vi "Read Type-Specific Macro Parameters.vi"(7 "Section":string, 8 "error in (no error)":errorcluster, 10 "Macro Step":T1, 11 "refnum":T5) -> (0 "error out":errorcluster, 2 "Macro Step out":T1={"Type"=enum."Mouse Move", "X"=0, "Y"=0, "Delay"=0, "Key"=65, "Repeat"=0, "RClick?"=FALSE, "App/Window Name"="", "Notes"="", "Assertion Type"=enum."Control Position", "Control Name"="", "Disabled"=enum."Enabled", "Visible"=enum."Visible", "Left"=0, "Top"=0, "Width"=0, "Height"=0, "Expected Image"={"image type"=0, "image depth"=0, "image"=[], "mask"=[], "colors"=[], "Rectangle"={"left"=0, "top"=0, "right"=0, "bottom"=0}}}, 3 "refnum out":T5)   [LabVIEW 2020, in "MacroAssert.lvlib"]
doc: "Reads the list of steps from macro config file defined by <B>refnum</B>."
uses:
  MacroAssert.lvlib
  <vilib>/ErrorRing/Error Ring.xnode
  <vilib>/Utility/config.llb/NI_LVConfig.lvlib
  <vilib>/Utility/config.llb/Read Key (String).vi
  <vilib>/Utility/config.llb/Read Key (I32).vi
  CTLs/Assertion Type.ctl
  <vilib>/Utility/error.llb/Error Cluster From Error Code.vi
  <vilib>/Utility/config.llb/Read Key (Boolean).vi
  <vilib>/Utility/config.llb/Read Key (U32).vi
  <vilib>/Utility/config.llb/Config Data RefNum.ctl
  CTLs/Step Type V3.ctl
  CTLs/Step V3.ctl
  <vilib>/picture/picture.llb/imagedata.ctl
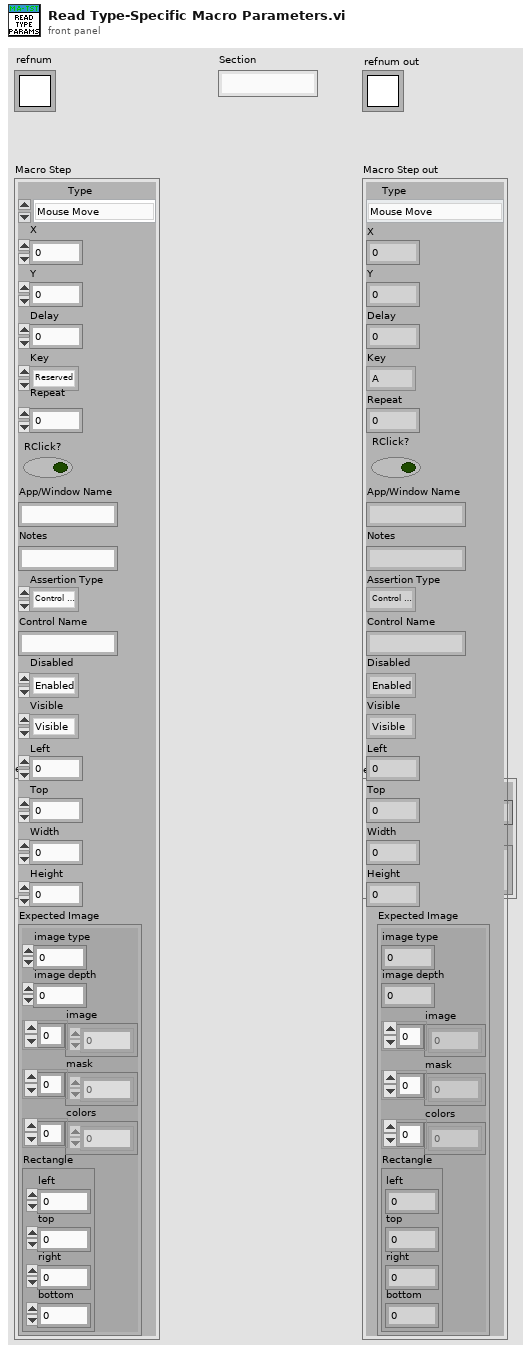
[diagram p1: front panel]
types:
  T1 = typedef "MacroAssert.lvlib/Step V3.ctl" = cluster{"Type":T2, "X":i32, "Y":i32, "Delay":i32, "Key":u8, "Repeat":i32, "RClick?":bool, "App/Window Name":string, "Notes":string, "Assertion Type":T3, "Control Name":string, "Disabled":enum8{"Enabled", "Disabled", "Disabled and Grayed Out"}, "Visible":enum16{"Visible", "Not Visible"}, "Left":i16, "Top":i16, "Width":i16, "Height":i16, "Expected Image":T4}
  T2 = typedef "MacroAssert.lvlib/Step Type V3.ctl" = enum16{"Mouse Move", "Mouse Click", "Key Press", "Wait", "Mouse Down", "Mouse Up", "Key Down", "Key Up", "Test Assertion", "Run Application", "Maximize Window", "Restore Window", "Minimize Window", "Close Window", "Bring Window to Front", "Send Window to Back"}
  T3 = typedef "MacroAssert.lvlib/Assertion Type.ctl" = enum16{"Control Position", "Control Visible", "Control Disabled", "Control Image"}
  T4 = typedef "imagedata.ctl" = cluster{"image type":i32, "image depth":i32, "image":u8[], "mask":u8[], "colors":u32[], "Rectangle":cluster{"left":i16, "top":i16, "right":i16, "bottom":i16}}
  T5 = typedef "NI_LVConfig.lvlib/Config Data RefNum.ctl" = refnum<k1>
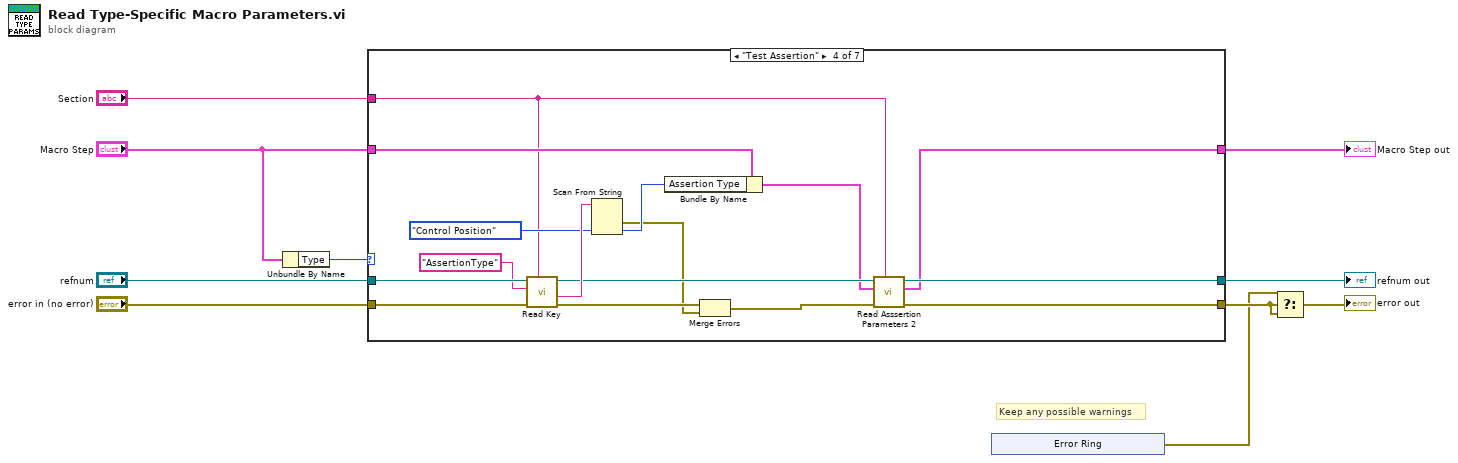
[diagram p0: block diagram]
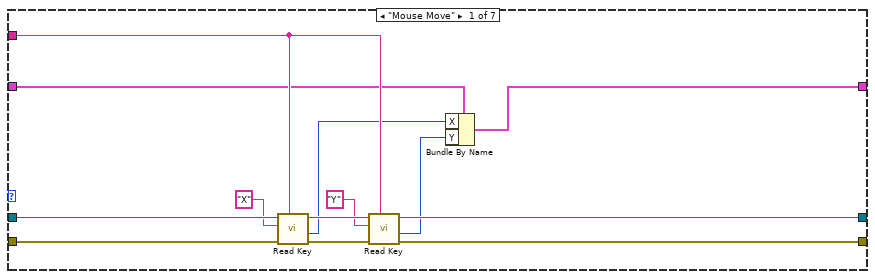
[diagram p2: hidden frame]
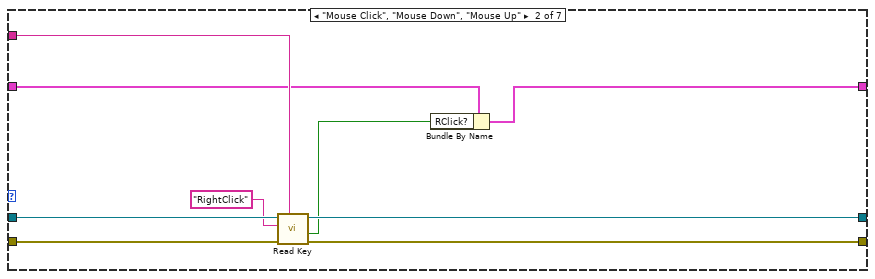
[diagram p3: hidden frame]
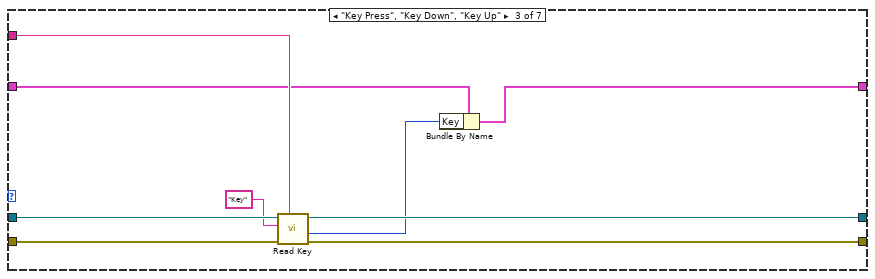
[diagram p4: hidden frame]
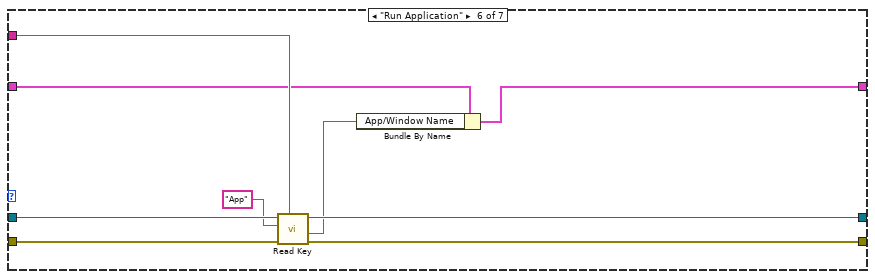
[diagram p6: hidden frame]
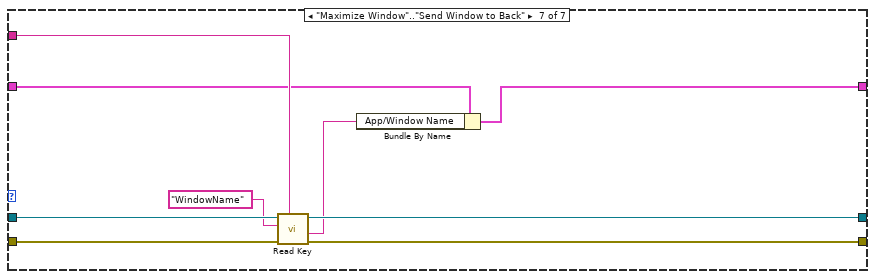
[diagram p7: hidden frame]
diagram:
  # "Keep any possible warnings"
  n1 = Unbundle By Name("Macro Step") -> ("Type"=w3:T2)
  n2 = case shown="\"Test Assertion\"" w3 {
    tunnel: "error in (no error)" -> [w23 w32 w41 w57 w60 w69 w78]
    tunnel: "refnum" -> [w19 w30 w39 w55 w59 w67 w76]
    tunnel: "Section" -> [w16 w28 w37 w47 _ w65 w74]
    tunnel: [w21 w31 w40 w43 w60 w68 w77] -> w10
    tunnel: [w15 w27 w35 w48 w59 w63 w72] -> w5
    tunnel: [w12 w24 w36 w45 w58 w64 w73] -> w4
    tunnel: "Macro Step" -> [w11 w25 w33 w53 w58 w61 w70]
    frame "Mouse Move" {
      n3 = call-poly <vilib>:"Read Key.vi"("section"=w16, "error in (no error)"=w23, "key"="X", "refnum"=w19) -> ("error out"=w22:errorcluster, "value"=w14:i32, "refnum out"=w20:T5)  [unwired: 4 in, 1 out]
      n4 = call-poly <vilib>:"Read Key.vi"("section"=w16, "error in (no error)"=w22, "key"="Y", "refnum"=w20) -> ("error out"=w21:errorcluster, "value"=w13:i32, "refnum out"=w15:T5)  [unwired: 4 in, 1 out]
      n5 = Bundle By Name(cluster=w11, "X"=w14, "Y"=w13) -> (w12:T1)
    }
    frame "Mouse Click", "Mouse Down", "Mouse Up" {
      n6 = call-poly <vilib>:"Read Key.vi"("section"=w28, "error in (no error)"=w32, "key"="RightClick", "refnum"=w30) -> ("error out"=w31:errorcluster, "value"=w26:bool, "refnum out"=w27:T5)  [unwired: 4 in, 1 out]
      n7 = Bundle By Name(cluster=w25, "RClick?"=w26) -> (w24:T1)
    }
    frame "Key Press", "Key Down", "Key Up" {
      n8 = call-poly <vilib>:"Read Key.vi"("section"=w37, "error in (no error)"=w41, "key"="Key", "refnum"=w39) -> ("error out"=w40:errorcluster, "value"=w34:u32, "refnum out"=w35:T5)  [unwired: 4 in, 1 out]
      n9 = Bundle By Name(cluster=w33, "Key"=w34) -> (w36:T1)
    }
    frame "Test Assertion" {
      n10 = call-poly <vilib>:"Read Key.vi"("section"=w47, "error in (no error)"=w57, "key"="AssertionType", "refnum"=w55) -> ("error out"=w56:errorcluster, "value"=w52:string, "refnum out"=w49:T5)  [unwired: 4 in, 1 out]
      n11 = Scan From String(input string=w52, default 1=Assertion_Type."Control Position" ("Assertion Type")) -> (error out=w42:errorcluster, output 1=w50:T3)  [unwired: 3 in, 2 out]
      n12 = Bundle By Name(cluster=w53, "Assertion Type"=w50) -> (w46:T1)
      n13 = Merge Errors(w56, w42) -> (w44:errorcluster)
      n14 = call "Read Asssertion Parameters 2.vi"("Section"=w47, "error in (no error)"=w44, "Macro Step"=w46, "refnum"=w49) -> ("error out"=w43:errorcluster, "Macro Step out"=w45:T1, "refnum out"=w48:T5)  [unwired: 5 in]
    }
    frame "Wait" {
    }
    frame "Run Application" {
      n15 = call-poly <vilib>:"Read Key.vi"("section"=w65, "error in (no error)"=w69, "key"="App", "refnum"=w67) -> ("error out"=w68:errorcluster, "value"=w62:string, "refnum out"=w63:T5)  [unwired: 4 in, 1 out]
      n16 = Bundle By Name(cluster=w61, "App/Window Name"=w62) -> (w64:T1)
    }
    frame "Maximize Window".."Send Window to Back" {
      n17 = call-poly <vilib>:"Read Key.vi"("section"=w74, "error in (no error)"=w78, "key"="WindowName", "refnum"=w76) -> ("error out"=w77:errorcluster, "value"=w71:string, "refnum out"=w72:T5)  [unwired: 4 in, 1 out]
      n18 = Bundle By Name(cluster=w70, "App/Window Name"=w71) -> (w73:T1)
    }
  }
  "refnum out" <- w5
  "Macro Step out" <- w4
  n19 = xnode "Error Ring"() -> ("error out"=w9:errorcluster)
  n20 = Select(t=w9, s=w10, f=w10) -> (s? t:f=→"error out":errorcluster)
